vi "Create spheres.vi"(2 "Render mode":T1(ring)=enum."Polygons", 3 "Colour":T2={"Red"=1.0, "Green"=0.0, "Blue"=0.0, "Alpha"=1.0}, 4 "Radius (model units)":sgl=1.0, 5 "Points array":sgl[][](array[numeric])) -> (0 "Error out":errorcluster, 1 "Points":refnum<vi>[](array[refnum]))   [LabVIEW 2014]
doc: "Use this VI to create an array of point objects to add to a render scene. These could be, for example, the point(s) of a collision."
uses:
  <vilib>/picture/3D Picture Control/Object/Create Object (drawable).vi
  <vilib>/picture/3D Picture Control/NI_3D Picture Control.lvlib
panel:
  # "PN 03/02/2015"
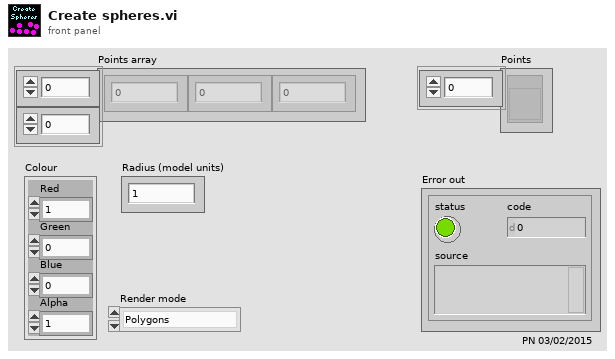
[diagram p1: front panel]
types:
  T1 = enum16{"Inherit Value", "Points", "Wireframe", "Polygons"}
  T2 = cluster{"Red":sgl, "Green":sgl, "Blue":sgl, "Alpha":sgl}
  T3 = enum16{"Inherit Value", "No Culling", "Cull Back Face", "Cull Front Face", "Cull Both Faces"}
  T4 = enum16{"Inherit Value", "Counterclockwise", "Clockwise"}
  T5 = cluster{"Numeric":sgl, "Numeric":sgl, "Numeric":sgl}
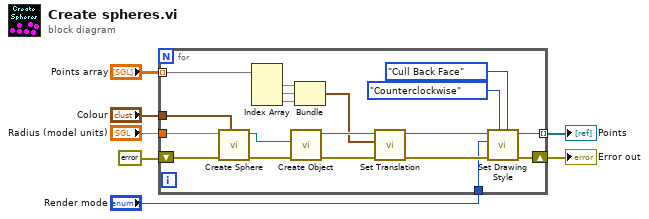
[diagram p0: block diagram]
diagram:
  n1 = for {
    tunnel: "Points array" -> [w15] mode=indexing
    shift-right: [w10] -> w3
    shift-left: errorcluster {"status"=FALSE, "code"=0, "source"=""} ("error in (no error)") -> [w13]
    tunnel: "Radius (model units)" -> [w12]
    tunnel: "Colour" -> [w11]
    tunnel: [w9] -> w2 mode=indexing
    tunnel: "Render mode" -> [w8]
    n2 = call <vilib>:"Create Sphere.vi"("Color"=w11, "error in (no error)"=w13, "Radius"=w12) -> ("error out"=w24:errorcluster, "New Sphere Refnum"=w23:refnum<vi>)  [unwired: 7 in]
    n3 = Index Array(array=w15) -> (element #1=w16:sgl, element #2=w17:sgl, element #3=w18:sgl)  [unwired: 3 in]
    n4 = call-poly <vilib>:"Create Object.vi"("error in (no error)"=w24, "Geometry"=w23) -> ("error out"=w22:errorcluster, "Scene:New Object"=w20:refnum<vi>)  [unwired: 8 in]
    n5 = Bundle("Numeric"=w16, "Numeric"=w17, "Numeric"=w18) -> (w14:T5)  [unwired: 1 in]
    n6 = call <vilib>:"Set Translation.vi"("error in (no error)"=w22, "Translation"=w14, "Scene Object"=w20) -> ("error out"=w21:errorcluster, "Translated Object"=w19:refnum<vi>)  [unwired: 7 in]
    n7 = call <vilib>:"Set Drawing Style.vi"("Face Culling Mode"=T3."Cull Back Face", "Frontface Mode"=T4."Counterclockwise", "error in (no error)"=w21, "Mode"=w8, "Scene Object In"=w19) -> ("error out"=w10:errorcluster, "Scene Object Out"=w9:refnum<vi>)  [unwired: 5 in]
  }
  "Error out" <- w3
  "Points" <- w2
